vi "simple tag.vi"() -> ()   [LabVIEW 2016]
uses:
  <vilib>/TagLibrary/Create Tag (Double).vi
  <vilib>/TagLibrary/Close Tag (Single).vi
  <vilib>/nisyscfg/Close (System).vi
  <vilib>/TagLibrary/TagLibrary.lvlib
  <vilib>/nisyscfg/nisyscfg.lvlib
panel:
  out "error out 2":errorcluster caption="error out"
  out "error out":errorcluster
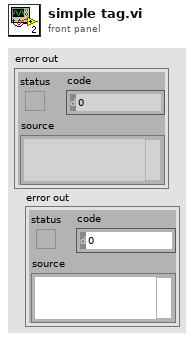
[diagram p1: front panel]
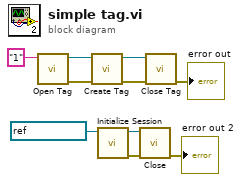
[diagram p0: block diagram]
diagram:
  n1 = call <vilib>:"Open Tag.vi"("tag path"="1" ("Tag")) -> ("error out"=w2:errorcluster, "tag reference out"=w5:refnum<k21>)  [unwired: 9 in]
  n2 = call-poly <vilib>:"Create Tag.vi"("error in (no error)"=w2, "tag reference in"=w5) -> ("error out"=w1:errorcluster, "tag reference out"=w4:refnum<k21>)  [unwired: 8 in]
  n3 = call <vilib>:"Initialize Session.vi"("Target (localhost)"=refnum<k21> "localhost") -> ("error out"=w8:errorcluster, "Session out"=w7:refnum<k21>)  [unwired: 9 in]
  n4 = call-poly <vilib>:"Close.vi"("error in (no error)"=w8, "Session in"=w7) -> ("error out"=→"error out 2":errorcluster)  [unwired: 9 in]
  n5 = call-poly <vilib>:"Close Tag.vi"("error in (no error)"=w1, "tag reference"=w4) -> ("error out"=→"error out":errorcluster)  [unwired: 9 in]
